vi "VariacMContoroller.vi"() -> ()   [LabVIEW 2019]
panel:
  in  "stop":bool
  out "Case":u32
  out "voltage higher":bool
  out "voltage lower":bool
  out "In Range?":bool
  in  "Tolearance in percentage":dbl
  in  "Voltage Feedback":dbl
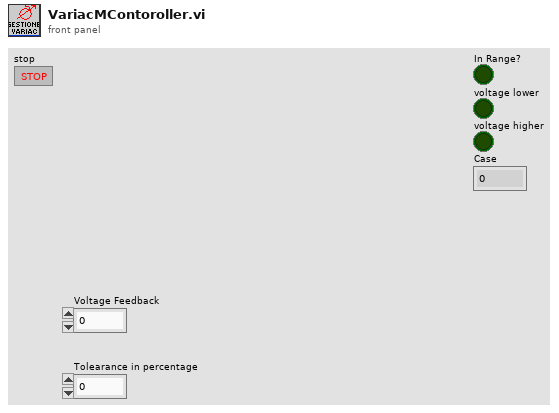
[diagram p1: front panel]
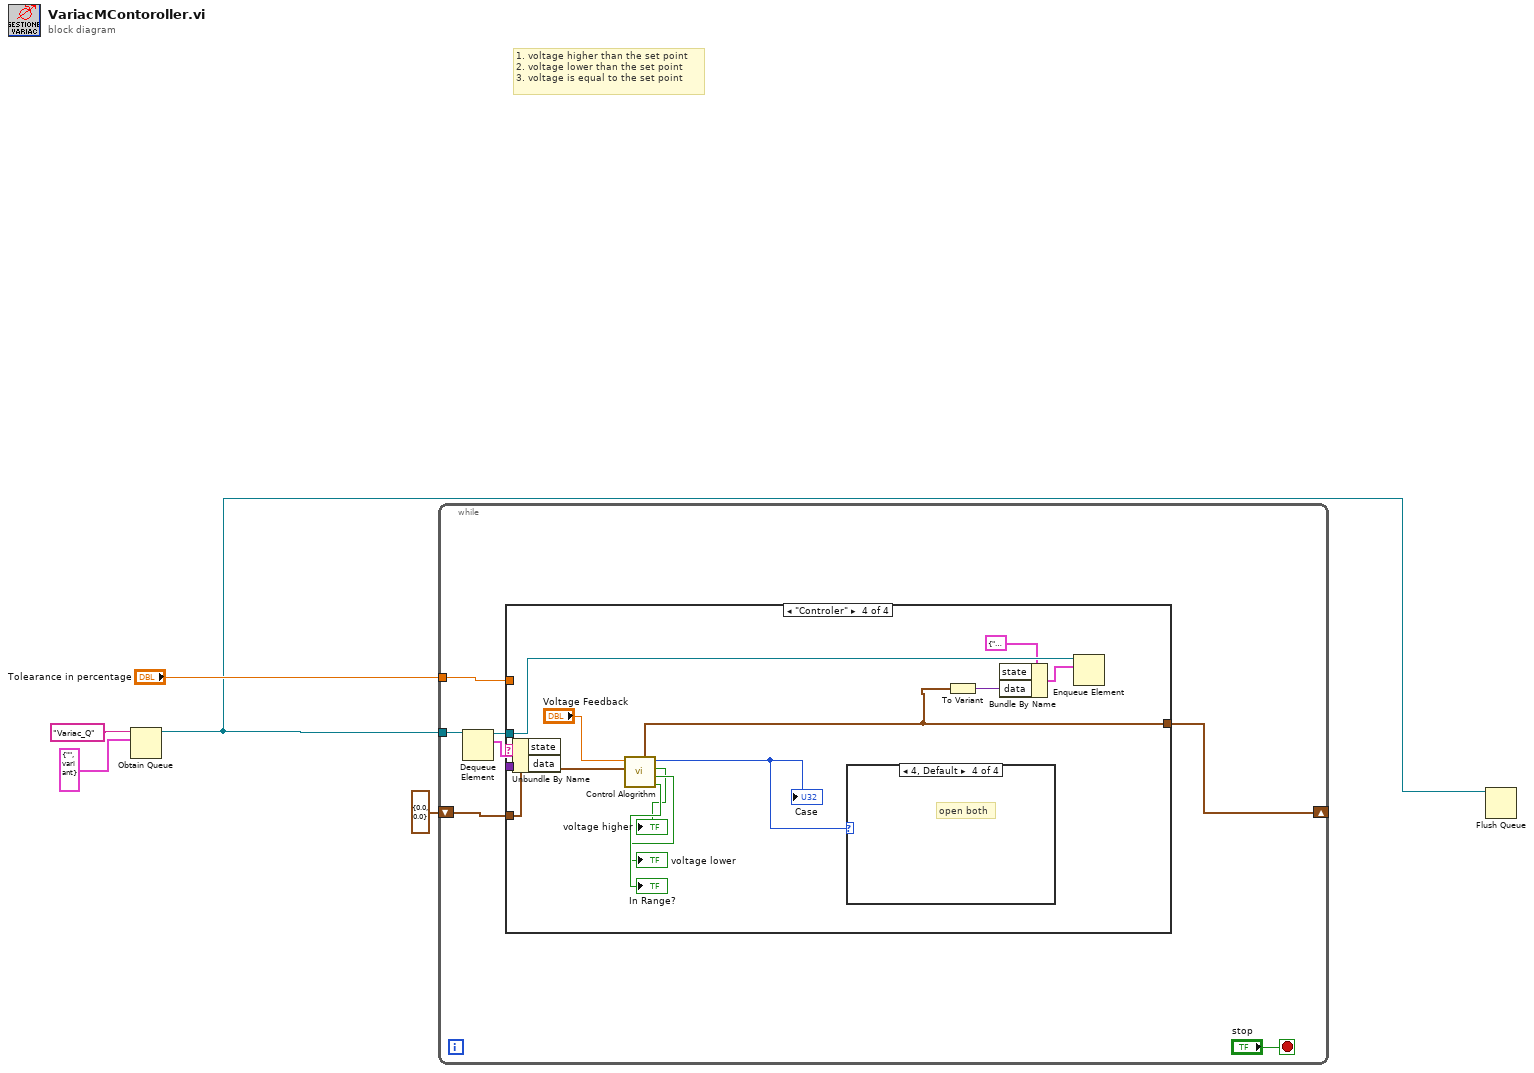
[diagram p0: block diagram]
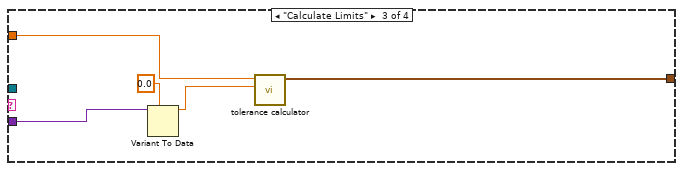
[diagram p4: hidden frame]
diagram:
  # "1. voltage higher than the set point \n2. voltage lower than the set point\n3. voltage is equal to the set point"
  n1 = Obtain Queue(name (unnamed)="Variac_Q", element data type=cluster{"state":string, "data":variant} {"state"="", "data"=variant} ("element")) -> (queue out=w1:refnum<queue>)  [unwired: 3 in, 2 out]
  n2 = while {
    tunnel: w1 -> [w14]
    tunnel: "Tolearance in percentage" -> [w10]
    shift-right: [w9] -> _
    shift-left: cluster{"upper limit":dbl, "lower limit":dbl} {"upper limit"=0.0, "lower limit"=0.0} ("output cluster") -> [w8]
    stop <- "stop" stop-if-true
    n3 = Dequeue Element(queue=w14) -> (queue out=w7:refnum<queue>, element=w13:cluster{"state":string, "data":variant})  [unwired: 2 in, 2 out]
    n4 = Unbundle By Name(w13) -> ("state"=w12:string, "data"=w11:variant)
    n5 = case shown="\"Controler\"" w12 {
      tunnel: w11 -> [_ _ w21 _]
      tunnel: w10 -> [_ _ w19 _]
      tunnel: [w15 w16 w17 w23] -> w9
      tunnel: w8 -> [w15 w16 _ w32]
      tunnel: w7 -> [_ _ _ w26]
      frame "Initalize", Default {
      }
      frame "Chuid Potenza Variac" {
        # "close Abilita ingresso variac \nclose Abilita ventilatore variac"
      }
      frame "Calculate Limits" {
        n6 = Variant To Data(type=0.0 ("Set point"), Variant=w21) -> (data=w18:dbl)  [unwired: 1 in, 1 out]
        n7 = call "tolerance calculator.vi"("Set point"=w18, "Tolerance"=w19) -> ("output cluster"=w17:cluster{"upper limit":dbl, "lower limit":dbl})  [unwired: 9 in]
      }
      frame "Controler" {
        n8 = call "Control Alogrithm.vi"("output cluster"=w32, "Voltage Feedback"="Voltage Feedback") -> ("In Range?"=→"In Range?":bool, "voltage lower"=→"voltage lower":bool, "voltage higher"=→"voltage higher":bool, "Case"=w27:u32, "output cluster 2"=w23:cluster{"upper limit":dbl, "lower limit":dbl})  [unwired: 5 in]
        "Case" <- w27
        n9 = case shown="4, Default" w27 {
          frame 0 {
          }
          frame 1 {
            # "Set Aumenta"
          }
          frame 2 {
            # "Set Diminuisci"
          }
          frame 4, Default {
            # "open both"
          }
        }
        n10 = To Variant(anything=w23) -> (Variant=w24:variant)
        n11 = Bundle By Name(cluster=cluster{"state":string, "data":variant} {"state"="", "data"=variant} ("element"), "data"=w24) -> (w22:cluster{"state":string, "data":variant})  [unwired: 1 in]
        n12 = Enqueue Element(queue=w26, element=w22) -> ()  [unwired: 2 in, 3 out]
      }
    }
  }
  n13 = Flush Queue(queue=w1) -> ()  [unwired: 1 in, 3 out]
